vi "Get FA Data.vi"(9 "Clust Refnum":refnum<vi>, 11 "FA Chosen Data Type":string) -> (0 "error out":errorcluster, 3 "ControlRefNums":refnum<vi>[](array[refnum]))   [LabVIEW 2016, in "M1M3SupportEUI_Views.lvlib"]
uses:
  M1M3SupportEUI_Views.lvlib
  Typedefs/FA Data And Events.ctl
  SALLV_m1m3/DataTypes/ForceActuatorData.ctl
  SALLV_m1m3/DataTypes/logevent_ForceActuatorForceWarning.ctl
  SALLV_m1m3/DataTypes/logevent_ForceActuatorInfo.ctl
  SALLV_m1m3/DataTypes/logevent_ForceActuatorState.ctl
  SALLV_m1m3/DataTypes/logevent_ForceActuatorWarning.ctl
  SALLV_m1m3/DataTypes/logevent_AppliedAberrationForces.ctl
  SALLV_m1m3/DataTypes/logevent_AppliedAccelerationForces.ctl
  SALLV_m1m3/DataTypes/logevent_AppliedActiveOpticForces.ctl
  SALLV_m1m3/DataTypes/logevent_AppliedAzimuthForces.ctl
  SALLV_m1m3/DataTypes/logevent_AppliedBalanceForces.ctl
  SALLV_m1m3/DataTypes/logevent_AppliedCylinderForces.ctl
  SALLV_m1m3/DataTypes/logevent_AppliedElevationForces.ctl
  SALLV_m1m3/DataTypes/logevent_AppliedForces.ctl
  SALLV_m1m3/DataTypes/logevent_AppliedOffsetForces.ctl
  SALLV_m1m3/DataTypes/logevent_AppliedStaticForces.ctl
  SALLV_m1m3/DataTypes/logevent_AppliedThermalForces.ctl
  SALLV_m1m3/DataTypes/logevent_AppliedVelocityForces.ctl
  SALLV_m1m3/DataTypes/logevent_RejectedAberrationForces.ctl
  SALLV_m1m3/DataTypes/logevent_RejectedAccelerationForces.ctl
  SALLV_m1m3/DataTypes/logevent_RejectedActiveOpticForces.ctl
  SALLV_m1m3/DataTypes/logevent_RejectedAzimuthForces.ctl
  SALLV_m1m3/DataTypes/logevent_RejectedBalanceForces.ctl
  SALLV_m1m3/DataTypes/logevent_RejectedCylinderForces.ctl
  SALLV_m1m3/DataTypes/logevent_RejectedElevationForces.ctl
  SALLV_m1m3/DataTypes/logevent_RejectedForces.ctl
  SALLV_m1m3/DataTypes/logevent_RejectedOffsetForces.ctl
  SALLV_m1m3/DataTypes/logevent_RejectedStaticForces.ctl
  SALLV_m1m3/DataTypes/logevent_RejectedThermalForces.ctl
  SALLV_m1m3/DataTypes/logevent_RejectedVelocityForces.ctl
  SALLV_m1m3/SALLV_m1m3.lvlib
  Typedefs/M1M3SupportEUI_TypeDefs.lvlib
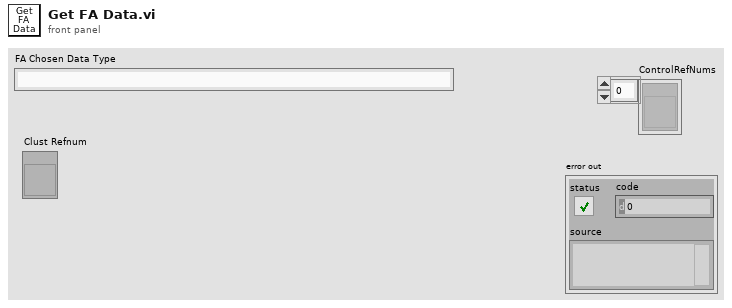
[diagram p1: front panel]
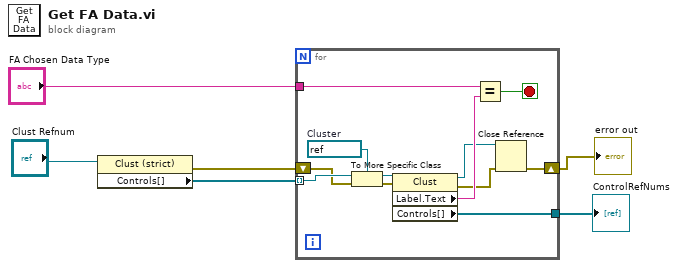
[diagram p0: block diagram]
diagram:
  n1 = property class="Clust (strict)"(reference="Clust Refnum") -> (error out=w2:errorcluster, "Controls[]"=w6:refnum<vi>[])  [unwired: 1 in, 1 out]
  n2 = for {
    tunnel: w6 -> [w18] mode=indexing
    tunnel: "FA Chosen Data Type" -> [w12]
    shift-right: [w8] -> w3
    shift-left: w2 -> [w17]
    tunnel: [w13] -> w4
    stop <- w10 stop-if-true
    w16 = refnum<vi> refnum  # Cluster
    n3 = To More Specific Class(target class=w16, reference=w18, error in=w17) -> (specific class reference=w15:refnum<vi>, error out=w14:errorcluster)
    n4 = property class="Clust"(reference=w15, error in=w14) -> (reference out=w7:refnum<vi>, error out=w9:errorcluster, "Label.Text"=w11:string, "Controls[]"=w13:refnum<vi>[])
    n5 = Equal?(x=w12, y=w11) -> (x = y?=w10:bool)
    n6 = Close Reference(reference=w7, error in (no error)=w9) -> (error out=w8:errorcluster)
  }
  "ControlRefNums" <- w4
  "error out" <- w3
